vi "CollectCopyrightNotices.vi"() -> ()   [LabVIEW 2020]
panel:
  out "error out":errorcluster
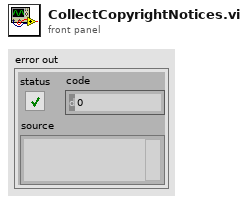
[diagram p1: front panel]
types:
  T1 = enum16{"open", "replace", "create", "open or create", "replace or create", "replace or create with confirmation"}
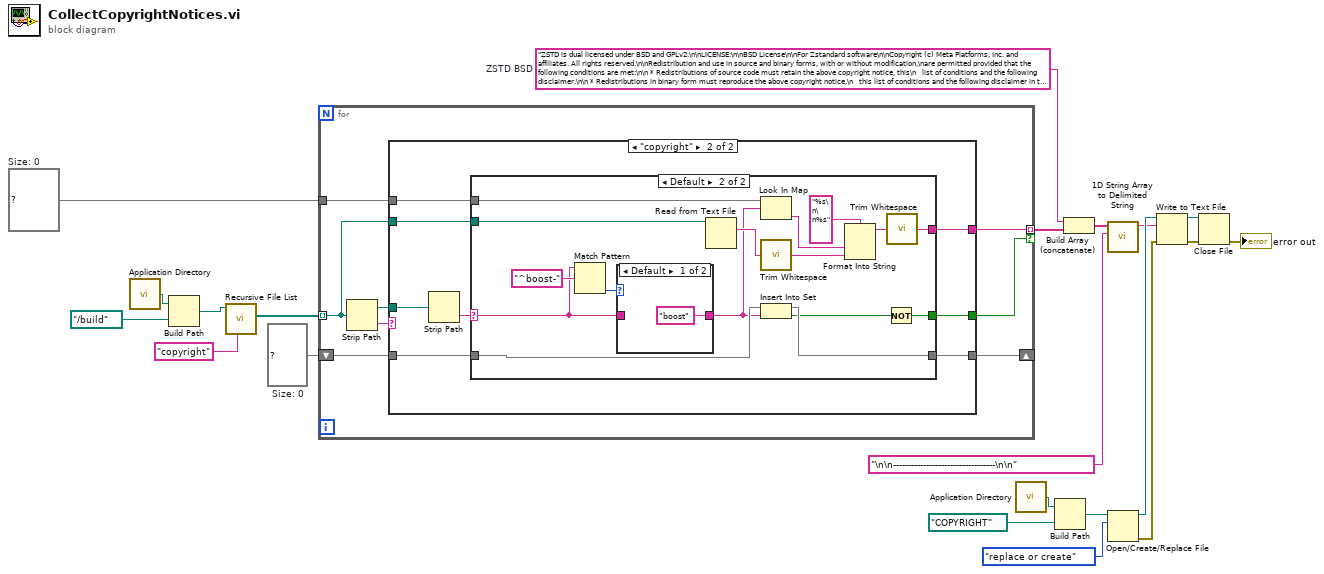
[diagram p0: block diagram]
diagram:
  w4 = set{string} {}  # Size: 0
  w5 = "ZSTD is dual licensed under BSD and GPLv2.\n\nLICENSE:\n\nBSD License\n\nFor Zstandard software\n\nCopyright (c) Meta Platforms, Inc. and affiliates. All rights reserved.\n\nRedistribution and use in source and binary forms, with or without modification,\nare permitted provided that the following conditions are met:\n\n * Redistributions of source code must retain the above copyright notice, this\n   list of conditions and the following disclaimer.\n\n * Redistributions in binary form must reproduce the above copyright notice,\n   this list of conditions and the following disclaimer in the documentation\n   and/or other materials provided with the distribution.\n\n * Neither the name Facebook, nor Meta, nor the names of its contributors may\n   be used to endorse or promote products derived from this software without\n   specific prior written permission.\n\nTHIS SOFTWARE IS PROVIDED BY THE COPYRIGHT HOLDERS AND CONTRIBUTORS \"AS IS\" AND\nANY EXPRESS OR IMPLIED WARRANTIES, INCLUDING, BUT NOT LIMITED TO, THE IMPLIED\nWARRANTIES OF MERCHANTABILITY AND FITNESS FOR A PARTICULAR PURPOSE ARE\nDISCLAIMED. IN NO EVENT SHALL THE COPYRIGHT HOLDER OR CONTRIBUTORS BE LIABLE FOR\nANY DIRECT, INDIRECT, INCIDENTAL, SPECIAL, EXEMPLARY, OR CONSEQUENTIAL DAMAGES\n(INCLUDING, BUT NOT LIMITED TO, PROCUREMENT OF SUBSTITUTE GOODS OR SERVICES;\nLOSS OF USE, DATA, OR PROFITS; OR BUSINESS INTERRUPTION) HOWEVER CAUSED AND ON\nANY THEORY OF LIABILITY, WHETHER IN CONTRACT, STRICT LIABILITY, OR TORT\n(INCLUDING NEGLIGENCE OR OTHERWISE) ARISING IN ANY WAY OUT OF THE USE OF THIS\nSOFTWARE, EVEN IF ADVISED OF THE POSSIBILITY OF SUCH DAMAGE."  # ZSTD BSD
  w20 = map{string, string} {}  # Size: 0
  n1 = call <vilib>:"Application Directory.vi"() -> ("Application Directory"=w2:path)
  n2 = Build Path(base path=w2, name or relative path=path "../build") -> (appended path=w3:path)
  n3 = call <vilib>:"Recursive File List.vi"("pattern"="copyright", "Folder Path"=w3) -> ("All Files in Dir"=w21:path[])  [unwired: 5 in, 4 out]
  n4 = for {
    tunnel: w21 -> [w27] mode=indexing
    tunnel: [w25] -> w6 mode=indexing if=w24
    tunnel: w20 -> [w26]
    shift-right: [w23] -> _
    shift-left: w4 -> [w22]
    n5 = Strip Path(path=w27) -> (stripped path=w28:path, name=w29:string)
    n6 = case shown="\"copyright\"" w29 {
      tunnel: w28 -> [_ w36]
      tunnel: w27 -> [_ w38]
      tunnel: w26 -> [_ w37]
      tunnel: [_ w34] -> w25
      tunnel: [_ w33] -> w24
      tunnel: [w30 w32] -> w23
      tunnel: w22 -> [w30 w31]
      frame Default {
      }
      frame "copyright" {
        n7 = Strip Path(path=w36) -> (name=w35:string)  [unwired: 1 out]
        n8 = case shown="Default" w35 {
          selector: w35 -> [_ w40]
          tunnel: w38 -> [_ w55]
          tunnel: w37 -> [_ w50]
          tunnel: [_ w48] -> w34
          tunnel: [_ w44] -> w33
          tunnel: [w39 w46] -> w32
          tunnel: w31 -> [w39 w47]
          frame "libiconv", "opencv4", "zstd" {
          }
          frame Default {
            n9 = Match Pattern(string=w40, regular expression="^boost-") -> (offset past match=w42:i32)  [unwired: 1 in, 3 out]
            n10 = case shown="Default" w42 {
              tunnel: ["boost" w57] -> w41
              tunnel: w40 -> [_ w57]
              frame Default {
              }
              frame -1 {
              }
            }
            n11 = Read from Text File(file (use dialog)=w55) -> (text=w54:string)  [unwired: 3 in, 3 out]
            n12 = Look In Map(map=w50, key=w41) -> (value=w49:string)  [unwired: 1 in, 1 out]
            n13 = call <vilib>:"Trim Whitespace.vi"("string"=w54) -> ("trimmed string"=w51:string)  [unwired: 1 in]
            n14 = Insert Into Set(10:w41, 11:w47) -> (2:w45:bool, 3:w46:set{string})
            n15 = Format Into String(format string="%s\n\n%s", w49, w51) -> (resulting string=w53:string)  [unwired: 2 in, 1 out]
            n16 = Not(x=w45) -> (.not. x?=w44:bool)
            n17 = call <vilib>:"Trim Whitespace.vi"("string"=w53) -> ("trimmed string"=w48:string)  [unwired: 1 in]
          }
        }
      }
    }
  }
  n18 = call <vilib>:"Application Directory.vi"() -> ("Application Directory"=w16:path)
  n19 = Build Path(base path=w16, name or relative path=path "COPYRIGHT") -> (appended path=w14:path)
  n20 = Build Array (concatenate)(w5, w6) -> (w18:string[])
  n21 = call <vilib>:"1D String Array to Delimited String.vi"("delimiter"="\n\n----------------------------------\n\n" ("string"), "string array"=w18) -> ("delimited string"=w8:string)  [unwired: 9 in]
  n22 = Open/Create/Replace File(file path (use dialog)=w14, operation (0:open)=T1."replace or create") -> (refnum out=w11:refnum<file>, error out=w12:errorcluster)  [unwired: 4 in, 1 out]
  n23 = Write to Text File(file (use dialog)=w11, text=w8, error in=w12) -> (refnum out=w9:refnum<file>, error out=w10:errorcluster)  [unwired: 1 in, 1 out]
  n24 = Close File(refnum=w9, error in=w10) -> (error out=→"error out":errorcluster)  [unwired: 1 out]
